vi "MoveBySteps.vi"(0 "TranslationStage in":refnum<class "KIM101.lvclass">, 1 "Direction":enum16{"Forward", "Backwards"}(ring)=enum."Backwards", 5 "Steps":dbl, 7 "Channel":u16(ring)=1 items=["Channel1"=1, "Channel2"=2, "Channel3"=3, "Channel4"=4], 9 "Speed":u32, 11 "error in (no error)":errorcluster, 13 "Polarity":enum16{"Positive", "Negative"}(ring)) -> (4 "TranslationStage out":refnum<class "KIM101.lvclass">, 15 "error out":errorcluster)   [LabVIEW 2023, in "TranslationStage Library.lvlib" / "KIM101.lvlib" / "KIM101.lvclass"]
uses:
  KIM101.lvclass
  C:/Program Files/National Instruments/LabVIEW 2023/vi.lib/ActorFramework/Actor/Actor.lvclass
  UIs/TranslationStage_UI/TranslationStage_UI/StageMoveDone_For_UI.ctl
  KIM101.lvclass/KIM101.ctl
  <vilib>/ActorFramework/Actor/Actor.lvclass/Actor.ctl
  Interfaces/AbstractInstrumentClasses/TranslationStages_LV/TranslationStagesComm Messages/StageMoveDone Msg/StageMoveDone Msg.lvclass/StageMoveDone Msg.ctl
  <vilib>/ActorFramework/Message Enqueuer/Message Enqueuer.lvclass/Message Enqueuer.ctl
  <vilib>/ActorFramework/Message Enqueuer/Enqueue.vi
  Interfaces/AbstractInstrumentClasses/TranslationStages_LV/TranslationStagesComm Messages/StageMoveDone Msg/StageMoveDone Msg.lvclass
  C:/Program Files/National Instruments/LabVIEW 2023/vi.lib/ActorFramework/Message/Message.lvclass
  <vilib>/ActorFramework/Message Priority Queue/Priority Enqueue.vi
  C:/Users/quantum/Documents/LVDAQ/Thorlabs.MotionControl.KCube.InertialMotorCLI.dll
  Thorlabs.MotionControl.KCube.InertialMotorCLI.dll
  <vilib>/ActorFramework/Actor/Actor.lvclass
  C:/Users/quantum/Documents/LVDAQ/ConcreteClasses/ConcreteInstrumentClasses/KIM101/KIM101/KIM101.lvclass
  C:/Users/quantum/Documents/LVDAQ/Interfaces/InitDeinitInterface/InitDeinit/InitDeinit.lvclass
  C:/Users/quantum/Documents/LVDAQ/Interfaces/AbstractInstrumentClasses/TranslationStages_LV/TranslationStageInterface/TranslationStagesInterface.lvclass
  typedefs/typedefs.lvlib
panel:
  in  "Positions":T1={"CH1 Pos"=0.0, "CH2 Pos"=0.0, "CH3 Pos"=0.0, "CH4 Pos"=0.0, "Home?"=TRUE}
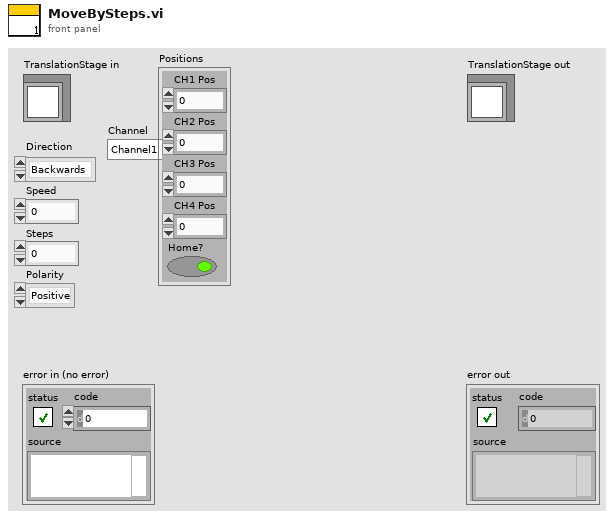
[diagram p1: front panel]
types:
  T1 = typedef "typedefs.lvlib/StageMoveDone_For_UI.ctl" = cluster{"CH1 Pos":sgl, "CH2 Pos":dbl, "CH3 Pos":dbl, "CH4 Pos":dbl, "Home?":bool}
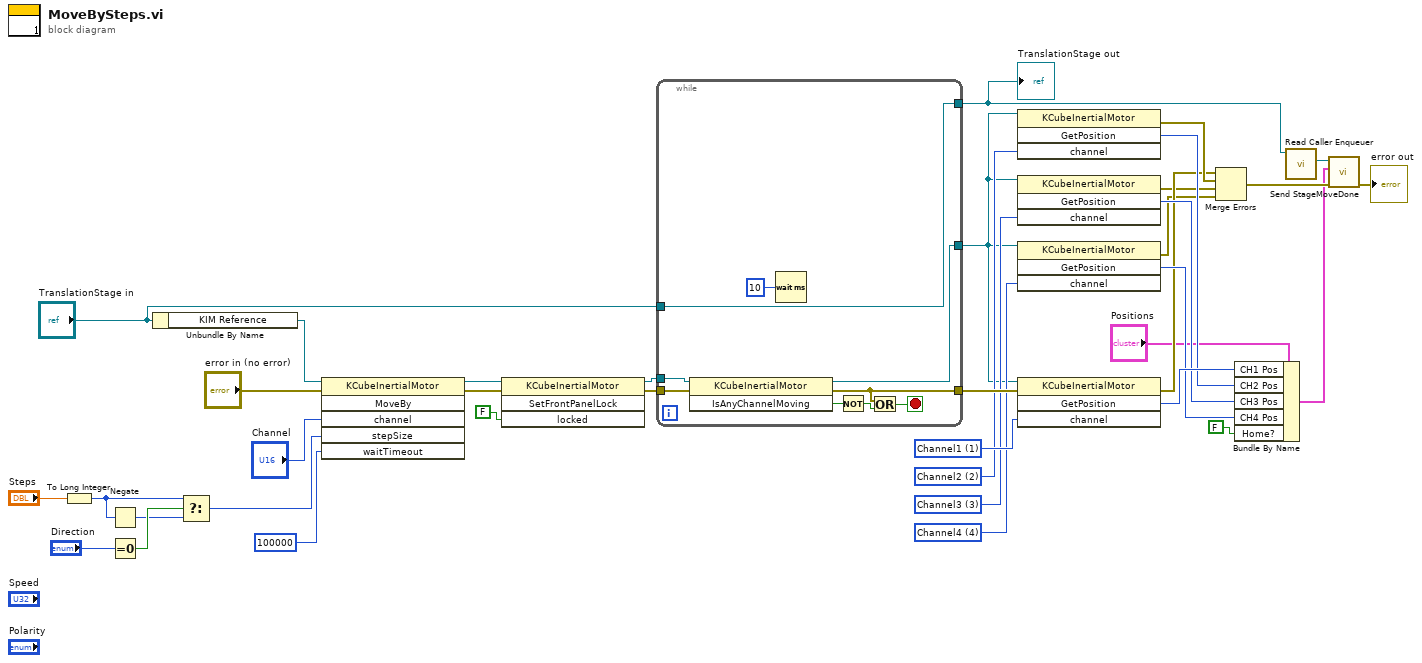
[diagram p0: block diagram]
diagram:
  w25 = 4 items=["Channel1"=1, "Channel2"=2, "Channel3"=3, "Channel4"=4] ("channel")
  w26 = 3 items=["Channel1"=1, "Channel2"=2, "Channel3"=3, "Channel4"=4] ("channel")
  w27 = 2 items=["Channel1"=1, "Channel2"=2, "Channel3"=3, "Channel4"=4] ("channel")
  w28 = 1 items=["Channel1"=1, "Channel2"=2, "Channel3"=3, "Channel4"=4] ("channel")
  n1 = To Long Integer(number="Steps") -> (32bit integer=w6:i32)
  n2 = Negate(x=w6) -> (-x=w8:i32)
  n3 = Equal To 0?(x="Direction") -> (x = 0?=w10:bool)
  n4 = Unbundle By Name("TranslationStage in") -> ("KIM Reference"=w33:refnum<k24>)
  n5 = Select(t=w6, s=w10, f=w8) -> (s? t:f=w7:i32)
  n6 = invoke class="KCubeInertialMotor" method="MoveBy"(reference=w33, error in="error in (no error)", "channel"="Channel", "stepSize"=w7, "waitTimeout"=100000) -> (reference out=w5:refnum<k24>, error out=w3:errorcluster)  [unwired: 1 in, 4 out]
  n7 = invoke class="KCubeInertialMotor" method="SetFrontPanelLock"(reference=w5, error in=w3, "locked"=FALSE) -> (reference out=w4:refnum<k24>, error out=w2:errorcluster)  [unwired: 1 in, 2 out]
  n8 = while {
    tunnel: [w43] -> w30
    tunnel: [w46] -> w34
    tunnel: "TranslationStage in" -> [w46]
    tunnel: w4 -> [w41]
    tunnel: w2 -> [w40]
    tunnel: [w38] -> w15
    stop <- w42 stop-if-true
    n9 = invoke class="KCubeInertialMotor" method="IsAnyChannelMoving"(reference=w41, error in=w40) -> (reference out=w38:refnum<k24>, error out=w43:errorcluster, "IsAnyChannelMoving"=w44:bool)  [unwired: 1 in]
    n10 = Wait (ms)(milliseconds to wait=u32 10) -> ()  [unwired: 1 out]
    n11 = Not(x=w44) -> (.not. x?=w39:bool)
    n12 = Or(x=w43, y=w39) -> (x .or. y?=w42:bool)
  }
  "TranslationStage out" <- w34
  n13 = invoke class="KCubeInertialMotor" method="GetPosition"(reference=w15, "channel"=w27) -> (error out=w20:errorcluster, "GetPosition"=w23:i32)  [unwired: 2 in, 2 out]
  n14 = invoke class="KCubeInertialMotor" method="GetPosition"(reference=w15, "channel"=w26) -> (error out=w17:errorcluster, "GetPosition"=w22:i32)  [unwired: 2 in, 2 out]
  n15 = invoke class="KCubeInertialMotor" method="GetPosition"(reference=w15, "channel"=w25) -> (error out=w16:errorcluster, "GetPosition"=w21:i32)  [unwired: 2 in, 2 out]
  n16 = invoke class="KCubeInertialMotor" method="GetPosition"(reference=w15, error in=w30, "channel"=w28) -> (error out=w19:errorcluster, "GetPosition"=w24:i32)  [unwired: 1 in, 2 out]
  n17 = Merge Errors(w19, w20, w17, w16) -> (w18:errorcluster)
  n18 = Bundle By Name(cluster="Positions", "CH1 Pos"=w24, "CH2 Pos"=w23, "CH3 Pos"=w22, "CH4 Pos"=w21, "Home?"=FALSE) -> (w14:T1)
  n19 = call <vilib>:"Read Caller Enqueuer.vi"("Actor"=w34) -> ("Caller Enqueuer"=w36:refnum<class "Message Enqueuer.lvclass">)  [unwired: 10 in]
  n20 = call "Send StageMoveDone.vi"("error in (no error)"=w18, "Positions"=w14, "Message Enqueuer"=w36) -> ("error out"=→"error out":errorcluster)  [unwired: 7 in, 1 out]
